vi "Tree Value Change.vi"(10 "Tree Data":cluster{"Tag":string[], "Settings":T1[]} {"Settings"."Data Type" items=["Tree Parent"=-1, "Numeric"=0, "String"=1, "Boolean"=2, "Enum"=3]}, 11 "Init Refs":T3) -> (3 "Value":string)   [LabVIEW 2020, in "Sequencer with Output Values.lvlib" / "Sequencer with Output Values.lvclass"]
uses:
  Sequencer with Output Values.lvclass
  Control Refs.ctl
  Tree Item Settings.ctl
  Data Type.ctl
  <vilib>/Utility/miscctls.llb/LVPositionTypeDef.ctl
  Data Type Enum.ctl
  Global Tree Data.vi
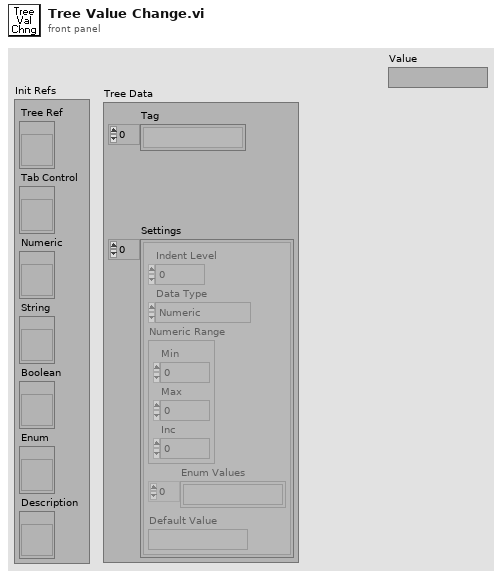
[diagram p1: front panel]
types:
  T1 = typedef "Sequencer with Output Values.lvlib/Sequencer with Output Values.lvclass/Tree Item Settings.ctl" = cluster{"Indent Level":i32, "Data Type":T2, "Numeric Range":cluster{"Min":dbl, "Max":dbl, "Inc":dbl}, "Enum Values":string[], "Default Value":string}
  T2 = typedef "Sequencer with Output Values.lvlib/Sequencer with Output Values.lvclass/Data Type.ctl" = i16
  T3 = typedef "Sequencer with Output Values.lvlib/Sequencer with Output Values.lvclass/Control Refs.ctl" = cluster{"Tree Ref":refnum<vi>, "Tab Control":refnum<vi>, "Numeric":refnum<vi>, "String":refnum<vi>, "Boolean":refnum<vi>, "Enum":refnum<vi>, "Description":refnum<vi>}
  T4 = typedef "LVPositionTypeDef.ctl" = cluster{"Left":i32, "Top":i32}
  T5 = typedef "Sequencer with Output Values.lvlib/Sequencer with Output Values.lvclass/Data Type Enum.ctl" = enum16{"Numeric", "String", "Boolean", "Enum"}
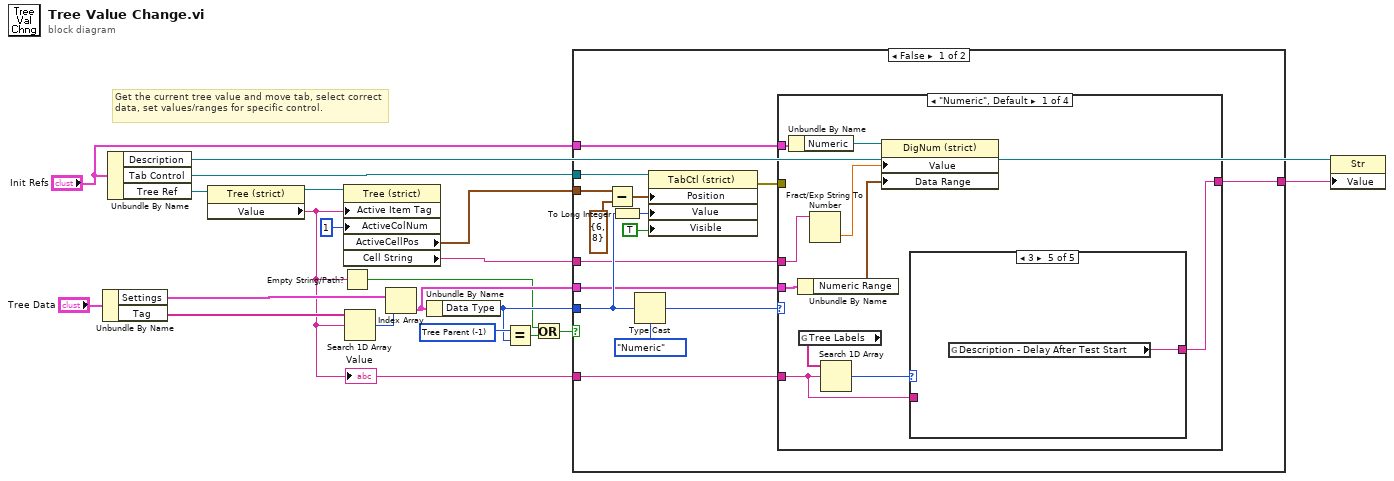
[diagram p0: block diagram]
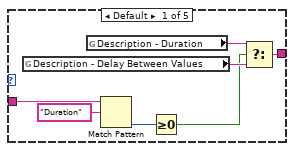
[diagram p2: hidden frame]
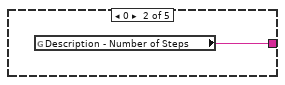
[diagram p3: hidden frame]
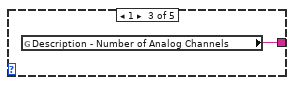
[diagram p4: hidden frame]
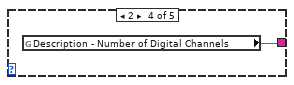
[diagram p5: hidden frame]
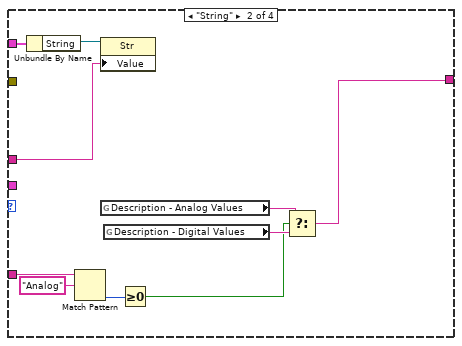
[diagram p6: hidden frame]
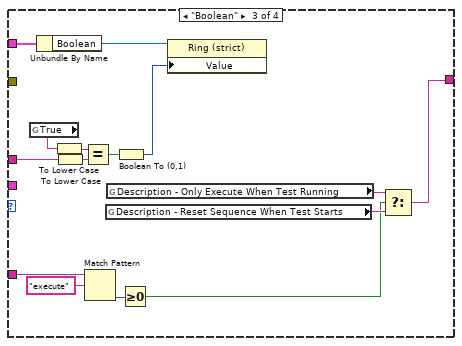
[diagram p7: hidden frame]
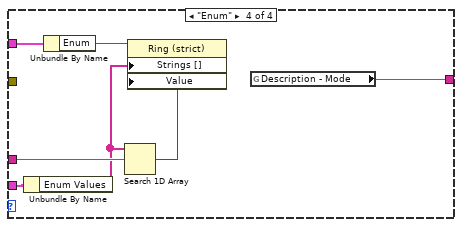
[diagram p8: hidden frame]
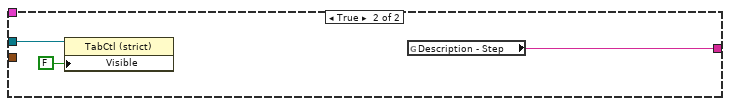
[diagram p9: hidden frame]
diagram:
  w11 = T2 -1 items=["Tree Parent"=-1, "Numeric"=0, "String"=1, "Boolean"=2, "Enum"=3, "Command"=4, "Numeric Min/Max"=5] ("Data Type")
  # "Get the current tree value and move tab, select correct data, set values/ranges for specific control."
  n1 = Unbundle By Name("Tree Data") -> ("Settings"=w13:T1[], "Tag"=w14:string[])
  n2 = Unbundle By Name("Init Refs") -> ("Description"=w3:refnum<vi>, "Tab Control"=w17:refnum<vi>, "Tree Ref"=w20:refnum<vi>)
  n3 = property class="Tree (strict)"(reference=w20) -> (reference out=w19:refnum<vi>, "Value"=w1:string)  [unwired: 1 in, 1 out]
  "Value" <- w1
  n4 = Empty String/Path?(string/path=w1) -> (empty?=w5:bool)
  n5 = property class="Tree (strict)"(reference=w19, "Active Item Tag"=w1, "ActiveColNum"=1 ("Active Cell:Active Column Number")) -> ("ActiveCellPos"=w16:T4, "Cell String"=w9:string)  [unwired: 1 in, 2 out]
  n6 = Search 1D Array(1D array=w14, element=w1) -> (index of element=w12:i32)  [unwired: 1 in]
  n7 = Index Array(array=w13, index=w12) -> (element=w8:T1)
  n8 = Unbundle By Name(w8) -> ("Data Type"=w7:T2)
  n9 = Equal?(x=w11, y=w7) -> (x = y?=w6:bool)
  n10 = Or(x=w5, y=w6) -> (x .or. y?=w4:bool)
  n11 = case shown="False" w4 {
    tunnel: w17 -> [w35 w91]
    tunnel: w16 -> [w32 _]
    tunnel: w7 -> [w29 _]
    tunnel: "Init Refs" -> [w25 _]
    tunnel: w9 -> [w24 _]
    tunnel: w8 -> [w23 _]
    tunnel: [w22 w89] -> w2
    tunnel: w1 -> [w21 _]
    frame False {
      n12 = Subtract(x=w32, y=T4 {"Left"=6, "Top"=8}) -> (x-y=w31:T4)
      n13 = To Long Integer(number=w29) -> (32bit integer=w34:i32)
      n14 = Type Cast(type=Data_Type_Enum."Numeric" ("Data Type"), x=w29) -> (*(type *) &x=w27:T5)
      n15 = property class="TabCtl (strict)"(reference=w35, "Position"=w31, "Value"=w34, "Visible"=TRUE) -> (error out=w26:errorcluster)  [unwired: 1 in, 1 out]
      n16 = case shown="\"Numeric\", Default" w27 {
        tunnel: w26 -> [_ _ _ _]
        tunnel: w25 -> [w45 w66 w81 w88]
        tunnel: w24 -> [w42 w64 w79 w85]
        tunnel: w23 -> [w43 _ _ w86]
        tunnel: [w37 w57 w71 w82] -> w22
        tunnel: w21 -> [w36 w61 w70 _]
        frame "Numeric", Default {
          n17 = Unbundle By Name(w45) -> ("Numeric"=w44:refnum<vi>)
          n18 = Unbundle By Name(w43) -> ("Numeric Range"=w40:cluster{"Min":dbl, "Max":dbl, "Inc":dbl})
          n19 = global read "Global Tree Data.vi" "Tree Labels"() -> (w39:string[])
          n20 = Fract/Exp String To Number(string=w42) -> (number=w41:dbl)  [unwired: 3 in, 1 out]
          n21 = Search 1D Array(1D array=w39, element=w36) -> (index of element=w38:i32)  [unwired: 1 in]
          n22 = property class="DigNum (strict)"(reference=w44, "Value"=w41, "Data Range"=w40) -> ()  [unwired: 1 in, 2 out]
          n23 = case shown="3" w38 {
            tunnel: [w46 w53 w54 w55 w56] -> w37
            tunnel: w36 -> [w51 _ _ _ _]
            frame Default {
              n24 = global read "Global Tree Data.vi" "Description - Delay Between Values"() -> (w48:string)
              n25 = global read "Global Tree Data.vi" "Description - Duration"() -> (w49:string)
              n26 = Match Pattern(string=w51, regular expression="Duration") -> (offset past match=w50:i32)  [unwired: 1 in, 3 out]
              n27 = Greater Or Equal To 0?(x=w50) -> (x >= 0?=w47:bool)
              n28 = Select(t=w49, s=w47, f=w48) -> (s? t:f=w46:string)
            }
            frame 0 {
              n29 = global read "Global Tree Data.vi" "Description - Number of Steps"() -> (w53:string)
            }
            frame 1 {
              n30 = global read "Global Tree Data.vi" "Description - Number of Analog Channels"() -> (w54:string)
            }
            frame 2 {
              n31 = global read "Global Tree Data.vi" "Description - Number of Digital Channels"() -> (w55:string)
            }
            frame 3 {
              n32 = global read "Global Tree Data.vi" "Description - Delay After Test Start"() -> (w56:string)
            }
          }
        }
        frame "String" {
          n33 = Unbundle By Name(w66) -> ("String"=w65:refnum<vi>)
          n34 = Match Pattern(string=w61, regular expression="Analog") -> (offset past match=w59:i32)  [unwired: 1 in, 3 out]
          n35 = property class="Str"(reference=w65, "Value"=w64) -> ()  [unwired: 1 in, 2 out]
          n36 = global read "Global Tree Data.vi" "Description - Analog Values"() -> (w63:string)
          n37 = global read "Global Tree Data.vi" "Description - Digital Values"() -> (w62:string)
          n38 = Greater Or Equal To 0?(x=w59) -> (x >= 0?=w58:bool)
          n39 = Select(t=w63, s=w58, f=w62) -> (s? t:f=w57:string)
        }
        frame "Boolean" {
          n40 = global read "Global Tree Data.vi" "True"() -> (w75:string)
          n41 = Unbundle By Name(w81) -> ("Boolean"=w80:refnum<vi>)
          n42 = To Lower Case(string=w75) -> (all lower case string=w74:string)
          n43 = To Lower Case(string=w79) -> (all lower case string=w78:string)
          n44 = Equal?(x=w74, y=w78) -> (x = y?=w77:bool)
          n45 = Match Pattern(string=w70, regular expression="execute") -> (offset past match=w68:i32)  [unwired: 1 in, 3 out]
          n46 = global read "Global Tree Data.vi" "Description - Reset Sequence When Test Starts"() -> (w72:string)
          n47 = global read "Global Tree Data.vi" "Description - Only Execute When Test Running"() -> (w73:string)
          n48 = Boolean To (0,1)(Boolean=w77) -> (0, 1=w76:i16)
          n49 = Greater Or Equal To 0?(x=w68) -> (x >= 0?=w67:bool)
          n50 = property class="Ring (strict)"(reference=w80, "Value"=w76) -> ()  [unwired: 1 in, 2 out]
          n51 = Select(t=w73, s=w67, f=w72) -> (s? t:f=w71:string)
        }
        frame "Enum" {
          n52 = Unbundle By Name(w86) -> ("Enum Values"=w84:string[])
          n53 = Unbundle By Name(w88) -> ("Enum"=w87:refnum<vi>)
          n54 = Search 1D Array(1D array=w84, element=w85) -> (index of element=w83:i32)  [unwired: 1 in]
          n55 = property class="Ring (strict)"(reference=w87, "Strings []"=w84, "Value"=w83) -> ()  [unwired: 1 in, 2 out]
          n56 = global read "Global Tree Data.vi" "Description - Mode"() -> (w82:string)
        }
      }
    }
    frame True {
      n57 = property class="TabCtl (strict)"(reference=w91, "Visible"=FALSE) -> ()  [unwired: 1 in, 2 out]
      n58 = global read "Global Tree Data.vi" "Description - Step"() -> (w89:string)
    }
  }
  n59 = property class="Str"(reference=w3, "Value"=w2) -> ()  [unwired: 1 in, 2 out]
